vi "Call DLLs.vi"   [LabVIEW 2010]
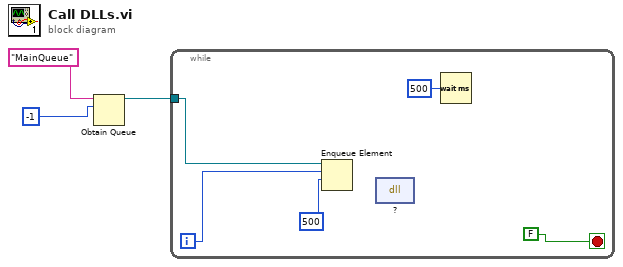
[diagram p0: block diagram]
diagram:
  n1 = Obtain Queue(name (unnamed)="MainQueue", element data type=-1 ("max queue size (-1, unlimited)")) -> (queue out=w1:refnum<queue>)  [unwired: 3 in, 2 out]
  n2 = while {
    tunnel: w1 -> [w7]
    i -> [w5]
    stop <- FALSE ("stop") stop-if-true
    n3 = Enqueue Element(queue=w7, element=w5, timeout in ms (-1)=500) -> ()  [unwired: 1 in, 3 out]
    n4 = dll-call lib="?" fn="?"() -> ()  [unwired: 4 in, 2 out]
    n5 = Wait (ms)(milliseconds to wait=u32 500) -> ()  [unwired: 1 out]
  }
